vi "rename channel.vi"(8 "error in":errorcluster, 9 "new name":string, 10 "old name":string, 11 "SHM configuration in":refnum<class "Shared Memory configuration.lvclass">) -> (0 "error out":errorcluster, 3 "SHM configuration out":refnum<class "Shared Memory configuration.lvclass">)   [LabVIEW 2013, in "Shared Memory configuration.lvclass"]
uses:
  module/configuration/Shared Memory configuration.lvclass
  module/configuration/Shared Memory configuration.lvclass/Shared Memory configuration.ctl
  <vilib>/NI/Tag Bus/tag/tag descriptor.lvclass/tag descriptor.ctl
  <vilib>/NI/Tag Bus/tag/read tag name.vi
  <vilib>/NI/Tag Bus Module Framework/channel/TBM channel.lvclass
  <vilib>/NI/Tag Bus/tag/tag descriptor.lvclass
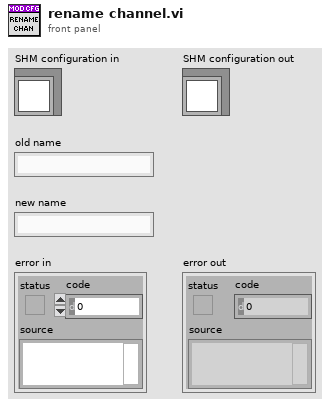
[diagram p1: front panel]
types:
  T1 = typedef "Shared Memory configuration.lvclass/Line.ctl" = cluster{"channel":refnum<class "TBM channel.lvclass">}
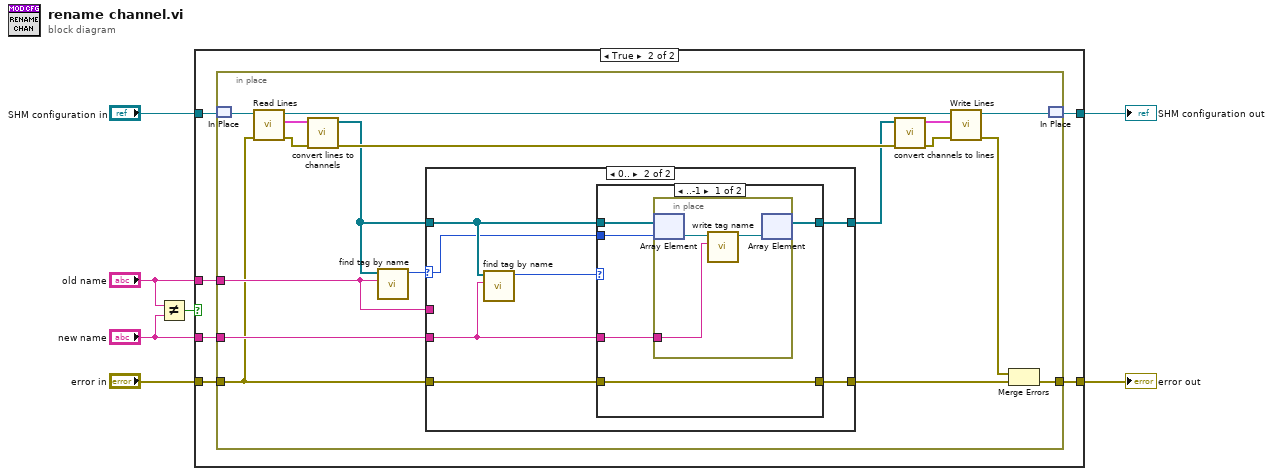
[diagram p0: block diagram]
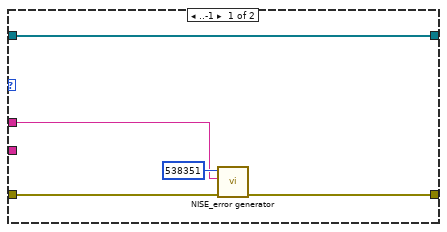
[diagram p3: hidden frame]
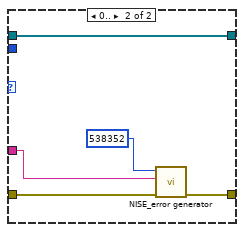
[diagram p4: hidden frame]
diagram:
  n1 = Not Equal?(x="old name", y="new name") -> (x != y?=w5:bool)
  n2 = case shown="True" w5 {
    tunnel: "error in" -> [w8 w15]
    tunnel: "SHM configuration in" -> [w9 w11]
    tunnel: [w9 w10] -> w6
    tunnel: [w8 w14] -> w1
    tunnel: "new name" -> [_ w13]
    tunnel: "old name" -> [_ w12]
    frame False {
    }
    frame True {
      n3 = in-place {
        in-place-border: w15 -> [w21]
        in-place-border: [w18] -> w14
        in-place-border: w13 -> [w32]
        in-place-border: w12 -> [w31]
        n4 = in-place-match #1(w11) -> (w27:refnum<class "Shared Memory configuration.lvclass">)
        n5 = call "Read Lines.vi"("error in"=w21, "Shared Memory configuration in"=w27) -> ("error out"=w29:errorcluster, "Lines"=w28:T1[], "Shared Memory configuration out"=w25:refnum<class "Shared Memory configuration.lvclass">)  [unwired: 7 in]
        n6 = call "convert lines to channels.vi"("error in (no error)"=w29, "Lines in"=w28) -> ("error out"=w22:errorcluster, "channels out"=w16:refnum<class "TBM channel.lvclass">[])  [unwired: 8 in]
        n7 = call <vilib>:"find tag by name.vi"("name"=w31, "tags in"=w16) -> ("index"=w30:i32)  [unwired: 9 in]
        n8 = case shown="0.." w30 {
          selector: w30 -> [_ w38]
          tunnel: w16 -> [w34 w43]
          tunnel: w31 -> [w36 _]
          tunnel: [w35 w39] -> w19
          tunnel: [w34 w44] -> w17
          tunnel: w21 -> [w33 w40]
          tunnel: w32 -> [_ w42]
          frame ..-1 {
            n9 = call <vilib>:"NISE_error generator.vi"("error in"=w33, "append error message"=w36, "error code (0)"=538351) -> ("error out"=w35:errorcluster)  [unwired: 6 in]
          }
          frame 0.. {
            n10 = call <vilib>:"find tag by name.vi"("name"=w42, "tags in"=w43) -> ("index"=w41:i32)  [unwired: 9 in]
            n11 = case shown="..-1" w41 {
              tunnel: [w49 w57] -> w44
              tunnel: w38 -> [w48 _]
              tunnel: w43 -> [w47 w57]
              tunnel: w42 -> [w46 w53]
              tunnel: w40 -> [w45 w55]
              tunnel: [w45 w56] -> w39
              frame ..-1 {
                n12 = in-place {
                  in-place-border: w46 -> [w50]
                  n13 = in-place-array #2(w47, w48) -> (w52:refnum<class "TBM channel.lvclass">)
                  n14 = call <vilib>:"write tag name.vi"("name"=w50, "system tag in"=w52) -> ("system tag out"=w51:refnum<class "TBM channel.lvclass">)  [unwired: 8 in, 1 out]
                  n15 = in-place-array #2(w51) -> (w49:refnum<class "TBM channel.lvclass">[])  [unwired: 1 out]
                }
              }
              frame 0.. {
                n16 = call <vilib>:"NISE_error generator.vi"("error in"=w55, "append error message"=w53, "error code (0)"=538352) -> ("error out"=w56:errorcluster)  [unwired: 6 in]
              }
            }
          }
        }
        n17 = call "convert channels to lines.vi"("error in (no error)"=w22, "channels"=w17) -> ("error out"=w23:errorcluster, "Lines"=w24:T1[])  [unwired: 8 in]
        n18 = call "Write Lines.vi"("error in (no error)"=w23, "Lines"=w24, "Shared Memory configuration in"=w25) -> ("error out"=w20:errorcluster, "Shared Memory configuration out"=w26:refnum<class "Shared Memory configuration.lvclass">)  [unwired: 7 in]
        n19 = Merge Errors(w20, w19) -> (w18:errorcluster)
        n20 = in-place-match #1(w26) -> (w10:refnum<class "Shared Memory configuration.lvclass">)
      }
    }
  }
  "error out" <- w1
  "SHM configuration out" <- w6
